vi "Update Object.vi"(6 "Transform":T1, 7 "Alpha":dbl, 9 "Alpha Blending Enabled":bool, 10 "Turntable Enabled":bool, 11 "Scene in":refnum<class "Scene.lvclass">) -> (3 "Scene out":refnum<class "Scene.lvclass">)   [LabVIEW 2022 SP3, in "Application.lvlib" / "Scene.lvclass"]
uses:
  Scene.lvclass
  Libraries/3D/Transform.ctl
  Libraries/3D/Vector 3D.ctl
  Scene.lvclass/Scene.ctl
  Libraries/3D/3D.lvlib
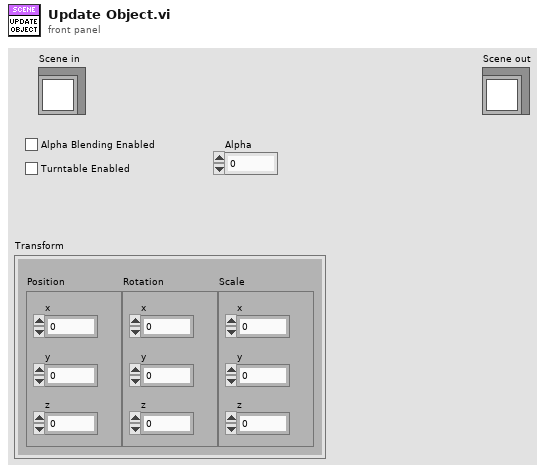
[diagram p1: front panel]
types:
  T1 = typedef "3D.lvlib/Transform.ctl" = cluster{"Position":T2, "Rotation":T2, "Scale":T2}
  T2 = typedef "3D.lvlib/Vector 3D.ctl" = cluster{"x":sgl, "y":sgl, "z":sgl}
  T3 = typedef "3D.lvlib/Object.ctl" = cluster{"Triangles":T4[], "Diffuse Colour":u32, "Transform":T1, "Name":string, "Alpha Blending Enabled":bool, "Alpha":dbl, "Turntable Enabled":bool}
  T4 = typedef "3D.lvlib/Triangle 3D.ctl" = cluster{"Point 1":T2, "Point 2":T2, "Point 3":T2}
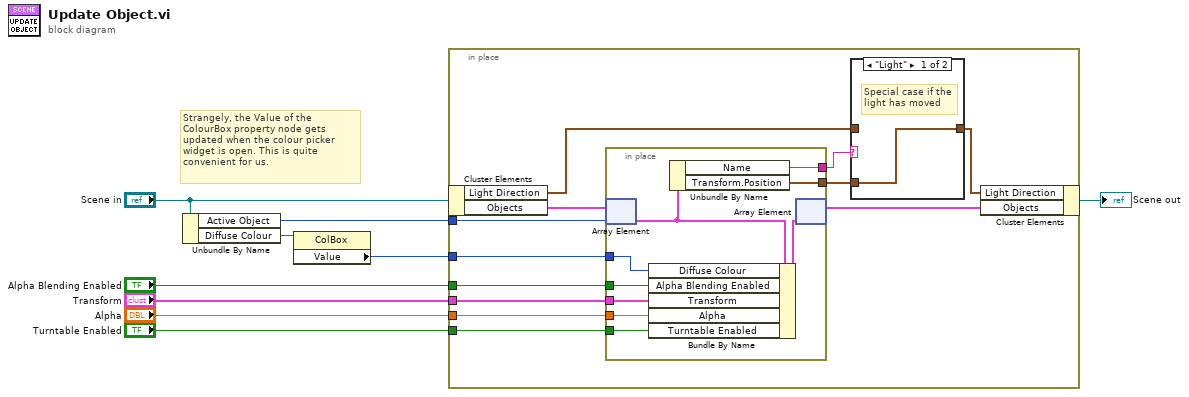
[diagram p0: block diagram]
diagram:
  # "Strangely, the Value of the ColourBox property node gets updated when the colour picker widget is open. This is quite convenient for us."
  n1 = Unbundle By Name("Scene in") -> ("Active Object"=w3:i32, "Diffuse Colour"=w4:refnum<vi>)
  n2 = property class="ColBox"(reference=w4) -> ("Value"=w2:u32)  [unwired: 1 in, 2 out]
  n3 = in-place {
    in-place-border: w3 -> [w20]
    in-place-border: "Transform" -> [w18]
    in-place-border: "Alpha Blending Enabled" -> [w17]
    in-place-border: "Alpha" -> [w16]
    in-place-border: w2 -> [w15]
    in-place-border: "Turntable Enabled" -> [w10]
    n4 = in-place-cluster #1("Scene in") -> ("Light Direction"=w12:T2, "Objects"=w21:T3[])
    n5 = in-place {
      in-place-border: w18 -> [w31]
      in-place-border: w17 -> [w30]
      in-place-border: w16 -> [w29]
      in-place-border: w15 -> [w28]
      in-place-border: [w26] -> w14
      in-place-border: [w25] -> w11
      in-place-border: w10 -> [w24]
      n6 = in-place-array #2(w21, w20) -> (w27:T3)
      n7 = Bundle By Name(cluster=w27, "Diffuse Colour"=w28, "Alpha Blending Enabled"=w30, "Transform"=w31, "Alpha"=w29, "Turntable Enabled"=w24) -> (w32:T3)
      n8 = Unbundle By Name(w27) -> ("Name"=w26:string, "Transform.Position"=w25:T2)
      n9 = in-place-array #2(w32) -> (w19:T3[])  [unwired: 1 out]
    }
    n10 = case shown="\"Light\"" w14 {
      tunnel: [w22 w23] -> w13
      tunnel: w12 -> [_ w23]
      tunnel: w11 -> [w22 _]
      frame "Light" {
        # "Special case if the light has moved"
      }
      frame Default {
      }
    }
    n11 = in-place-cluster #1("Light Direction"=w13, "Objects"=w19) -> (→"Scene out":refnum<class "Scene.lvclass">)
  }
